vi "Nan_Inf_replaced.vi"(1 "Value":dbl=2.0 format="%#_13g", 2 "IN with Inf and NaN":dbl[](array[numeric])) -> (0 "Out with NaN and Inf replaced":dbl[](array[numeric]))   [LabVIEW 2020]
uses:
  <userlib>/_OpenG.lib/array/array.llb/Search 1D Array (DBL)__ogtk.vi
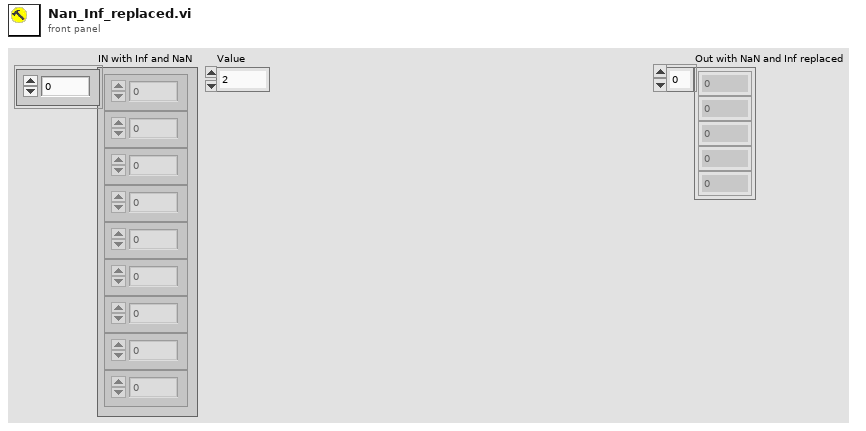
[diagram p1: front panel]
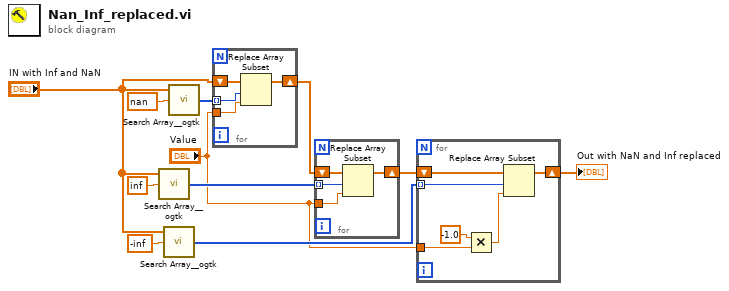
[diagram p0: block diagram]
diagram:
  n1 = call-poly <userlib>:"Search Array__ogtk.vi"("Array"="IN with Inf and NaN", "Element Data"=inf) -> ("Indices of Elements"=w7:i32[])  [unwired: 7 in]
  n2 = call-poly <userlib>:"Search Array__ogtk.vi"("Array"="IN with Inf and NaN", "Element Data"=-inf) -> ("Indices of Elements"=w6:i32[])  [unwired: 7 in]
  n3 = call-poly <userlib>:"Search Array__ogtk.vi"("Array"="IN with Inf and NaN", "Element Data"=nan) -> ("Indices of Elements"=w8:i32[])  [unwired: 7 in]
  n4 = for {
    tunnel: w8 -> [w15] mode=indexing
    shift-right: [w13] -> w5
    shift-left: "IN with Inf and NaN" -> [w14]
    tunnel: "Value" -> [w12]
    n5 = Replace Array Subset(array=w14, new element=w12, index=w15) -> (w13:dbl[])
  }
  n6 = for {
    tunnel: w7 -> [w17] mode=indexing
    shift-right: [w18] -> w4
    shift-left: w5 -> [w19]
    tunnel: "Value" -> [w16]
    n7 = Replace Array Subset(array=w19, new element=w16, index=w17) -> (w18:dbl[])
  }
  n8 = for {
    tunnel: w6 -> [w25] mode=indexing
    shift-right: [w23] -> w3
    shift-left: w4 -> [w24]
    tunnel: "Value" -> [w22]
    n9 = Multiply(x=-1.0, y=w22) -> (x*y=w21:dbl)
    n10 = Replace Array Subset(array=w24, new element=w21, index=w25) -> (w23:dbl[])
  }
  "Out with NaN and Inf replaced" <- w3
